vi "Shooter_Determiner.vi"() -> ()   [LabVIEW 2020]
uses:
  Subsystems/Cowl/Cowl_Cluster.ctl
  Subsystems/Cowl/Cowl_States.ctl
  <vilib>/Rock Robotics/WPI/DriverStation/WPI_DriverStationRobotMode2.ctl
  Subsystems/Flywheel/Flywheel_Cluster.ctl
  Subsystems/Flywheel/Flywheel_States.ctl
  Subsystems/Turret/Turret_Cluster.ctl
  Subsystems/Turret/Turret_States.ctl
  Shooter_Control_States.ctl
  Shooter_Cluster.ctl
  Globals/Turret_Globals.vi
  Globals/Flywheel_Globals.vi
  Globals/Cowl_Globals.vi
  Shooter_Globals.vi
  Robot Global Data.vi
  Globals/Sensor_Values.vi
panel:
  out "angle_to_target":dbl
  in  "Cowl_Puke_Goal_Angle":dbl=61.0
  in  "Flywheel_Puke_Velocity_Goal":dbl=1000.0
  in  "no_target_flywheel_velocity":dbl=3200.0
  in  "no_target_cowl_angle":dbl=61.0
  in  "disable turret auto_target":bool
  in  "use table in test":bool
  out "cowl_goal_angle":dbl=61.0
  out "Flywheel_Goal_Velocity":dbl=3200.0
  in  "use auto-target turret in test":bool
  in  "Cowl_Angle_Test_Goal":dbl=50.0
  in  "use front panel cowl goal":bool
  in  "use front panel flywheel velocity goal":bool
  in  "Flywheel_Velocity_Test_Goal":dbl=3500.0
  out "Limelight_Distance_To_Target (in)":dbl=124.83321913736278
  in  "Shooter_Table":dbl[][](array[numeric])=[[55.0, 3350.0, 60.0], [81.0, 3500.0, 54.0], [110.0, 3800.0, 50.0], [143.0, 4100.0, 45.0], [179.0, 4700.0, 43.0]]
  in  "Use Equation?":bool
  out "loop time":u32=31
  out "timed out?":bool=TRUE
  # "68    3800    61"
  # "distance | flywheel velocity | cowl angle"
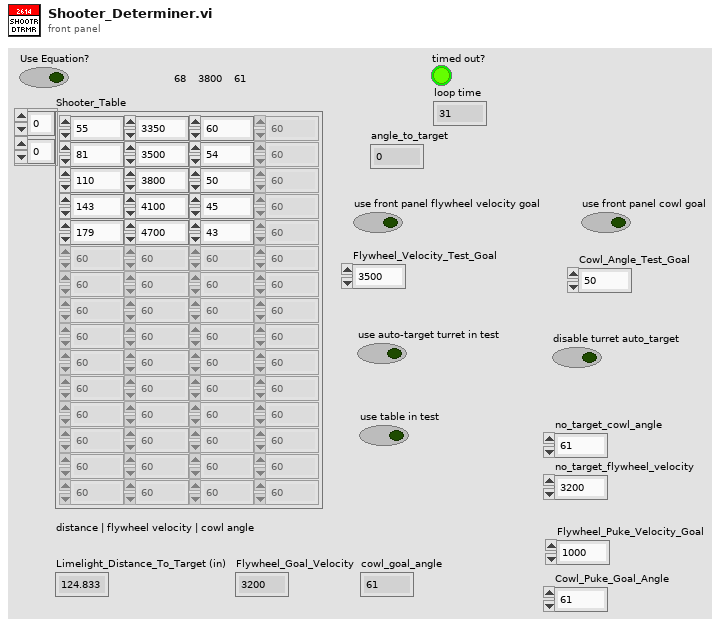
[diagram p1: front panel]
types:
  T1 = typedef "Shooter_Control_States.ctl" = enum16{"No-Op", "Limelight_Shooting", "Shoot_From_Pose", "Test", "Command_Shoot", "Manual", "Puke-Op", "Command_Shoot_From_Pose", "Turret Control", "Turret_Cowl_Zero"}
  T2 = typedef "Turret_Cluster.ctl" = cluster{"Turret_Control_State":T3, "Manual_Speed":dbl, "Step":i32, "Parameter_1":dbl, "Parameter_2":dbl, "Parameter_3":dbl, "Auto_Notifier":refnum<notifier>, "Goal_Angle":dbl, "Camera_Goal_X":dbl}
  T3 = typedef "Turret_States.ctl" = enum16{"Manual_Percent_Voltage", "Auto-Target", "Command_TurnToPosition", "Command_Auto_Target", "GoToZero", "No-Op", "Test_Position_Control", "Auto-Track"}
  T4 = typedef "Flywheel_Cluster.ctl" = cluster{"Flywheel_Throttle":dbl, "Flywheel_Control_State":T5, "Parameter_1":dbl, "Parameter_2":dbl, "Auto_Notifier":refnum<notifier>, "Step":dbl, "Flywheel_Velocity_Goal":dbl, "Flywheel_On ":bool}
  T5 = typedef "Flywheel_States.ctl" = enum16{"No-Op", "Percent_Voltage", "Speed_Control", "Speed_Control_Manual", "Command_SpinUp", "Command_SpinUpAuto"}
  T6 = typedef "WPI_DriverStationRobotMode2.ctl" = enum16{"Autonomous Disabled", "Autonomous Enabled", "Teleop Disabled", "Teleop Enabled", "Disconnected", "Finish", "Test Disabled", "Test Enabled", "Emergency Stopped"}
  T7 = typedef "Cowl_Cluster.ctl" = cluster{"Cowl_Control_State":T8, "Manual_Cowl_Throttle":dbl, "Cowl_Goal_Angle":dbl}
  T8 = typedef "Cowl_States.ctl" = enum16{"Manual_%VBus", "GoToAngle", "No-Op", "GoToZero"}
  T9 = typedef "Shooter_Cluster.ctl" = cluster{"Control_State":T1, "Shooting?":bool, "UpperGoal?":bool, "Limelight?":bool, "Flywheel_%Vbus":dbl, "Cowl_%Vbus":dbl, "Turret_%Vbus":dbl, "Parameters":dbl[], "Auto_Notifier":refnum<notifier>, "Step":i32, "Zero_Turret":bool, "Puke?":bool, "Turret_Target":dbl, "Turret_Control?":bool, "Turret_Manual_Control?":bool}
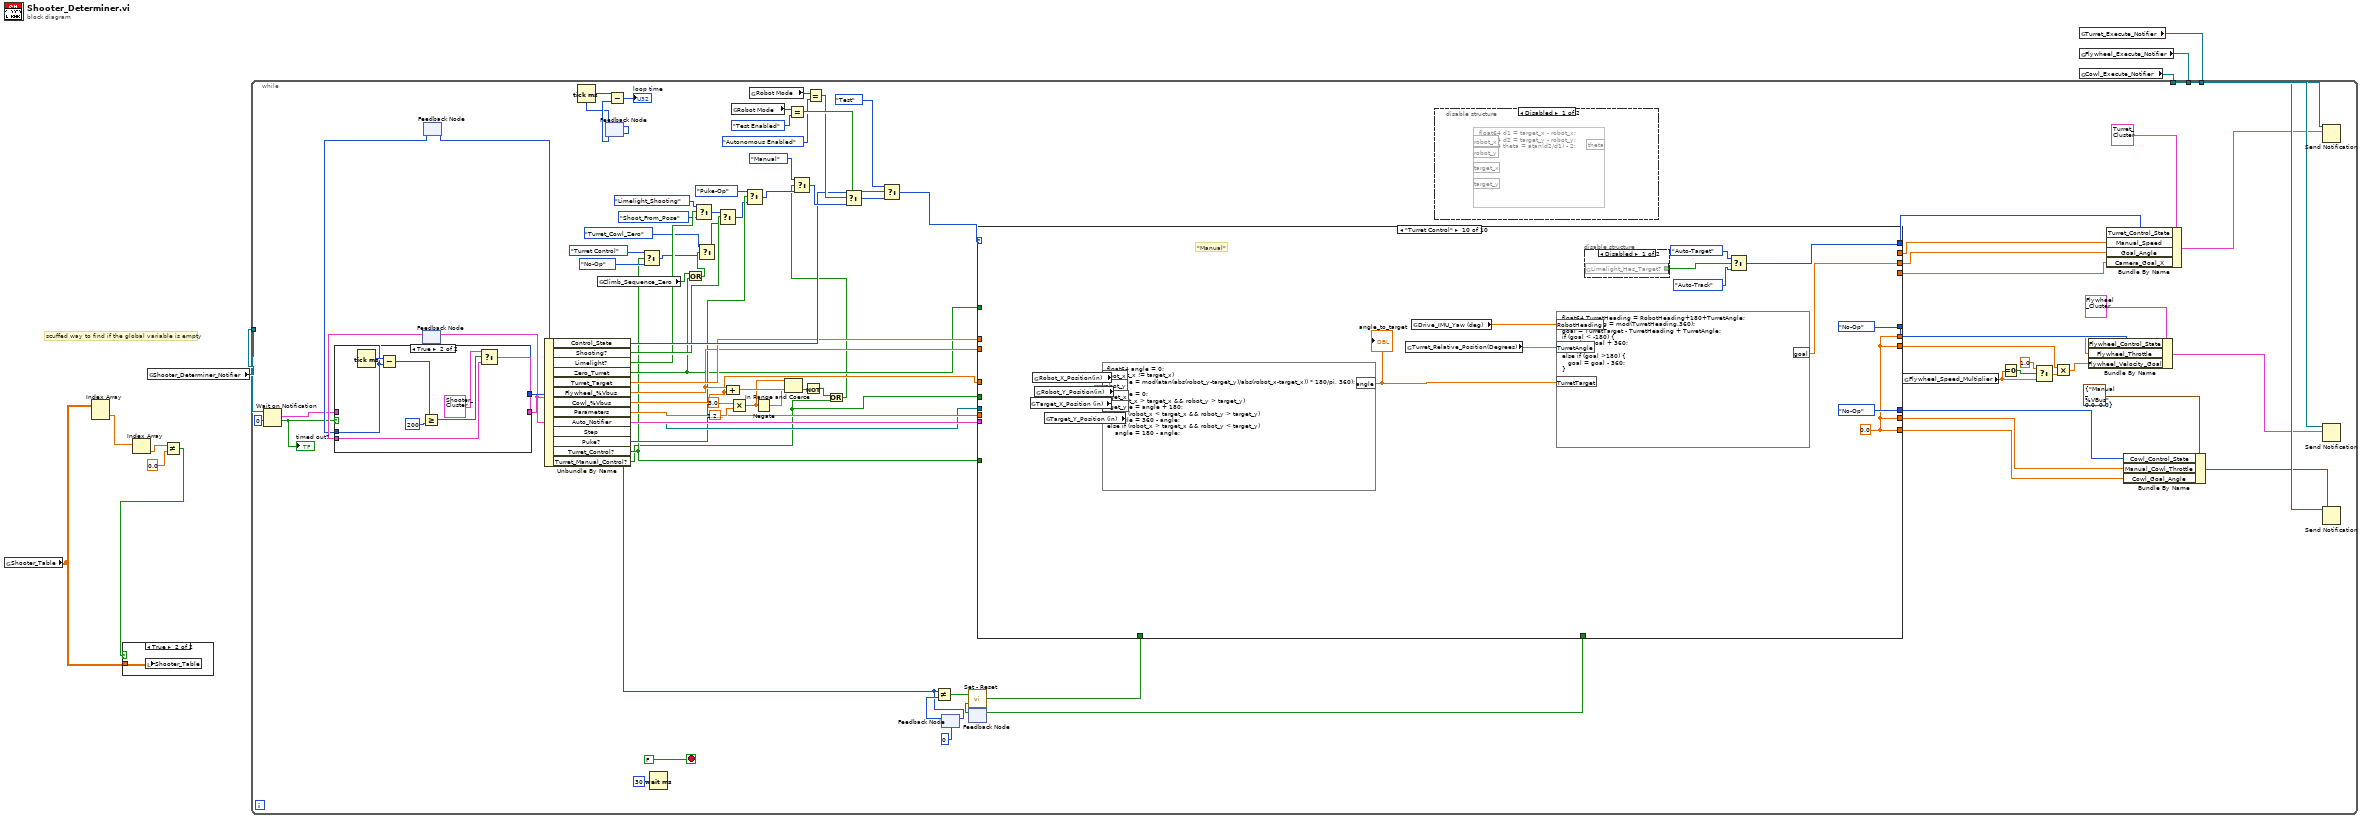
[diagram p0: block diagram]
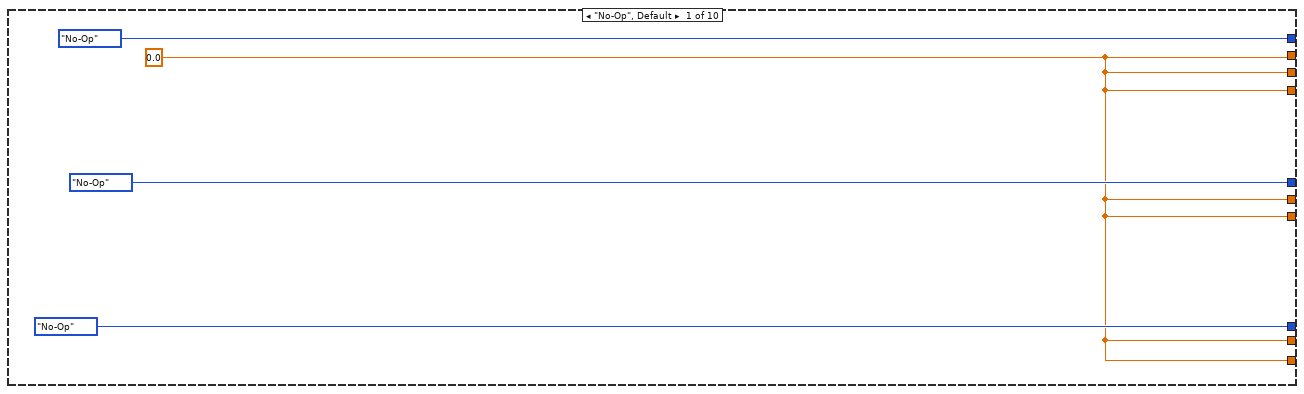
[diagram p4: hidden frame]
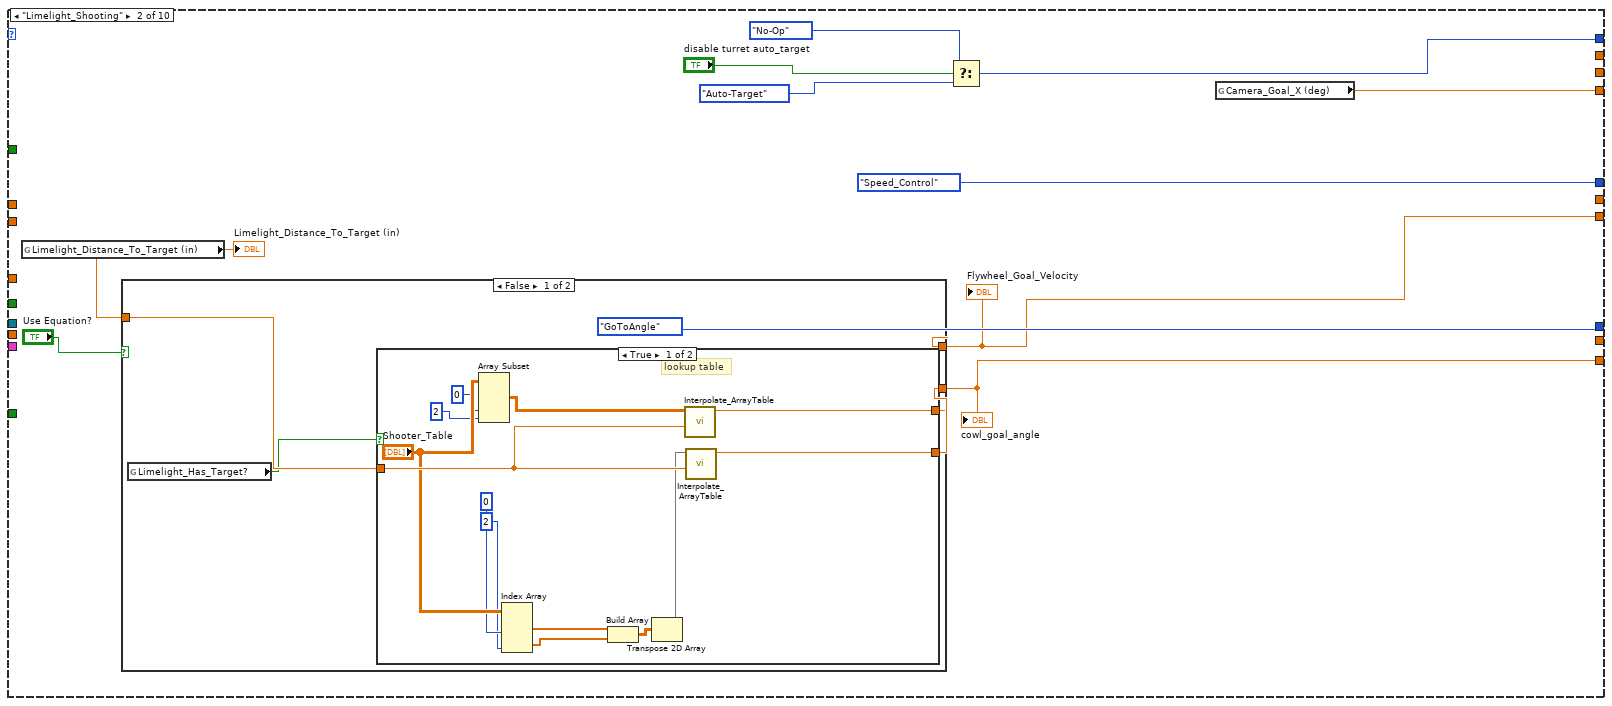
[diagram p5: hidden frame]
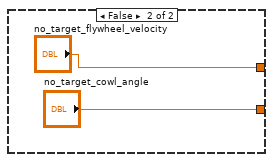
[diagram p6: hidden frame]
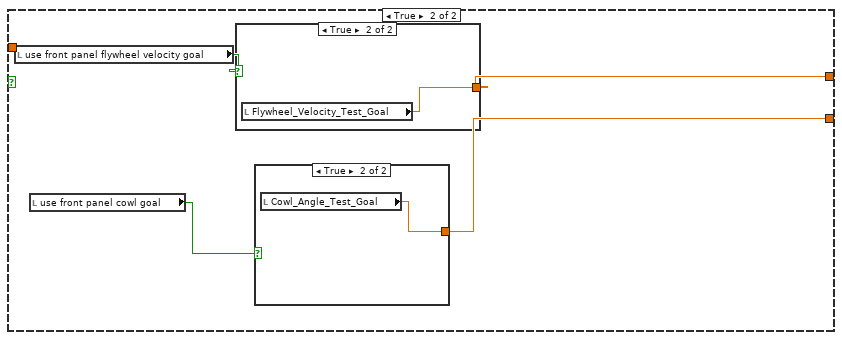
[diagram p7: hidden frame]
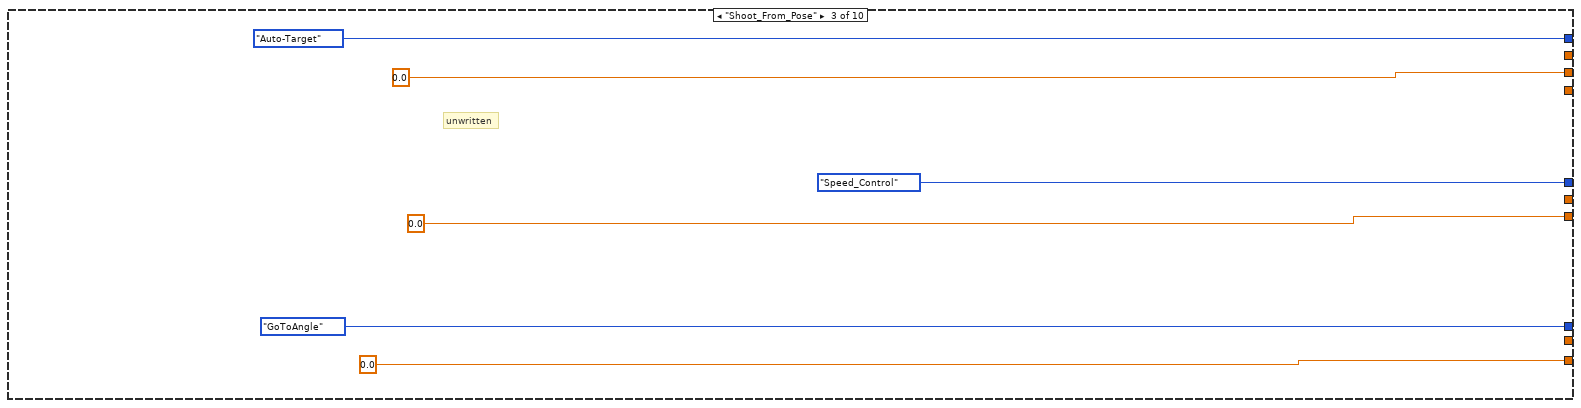
[diagram p10: hidden frame]
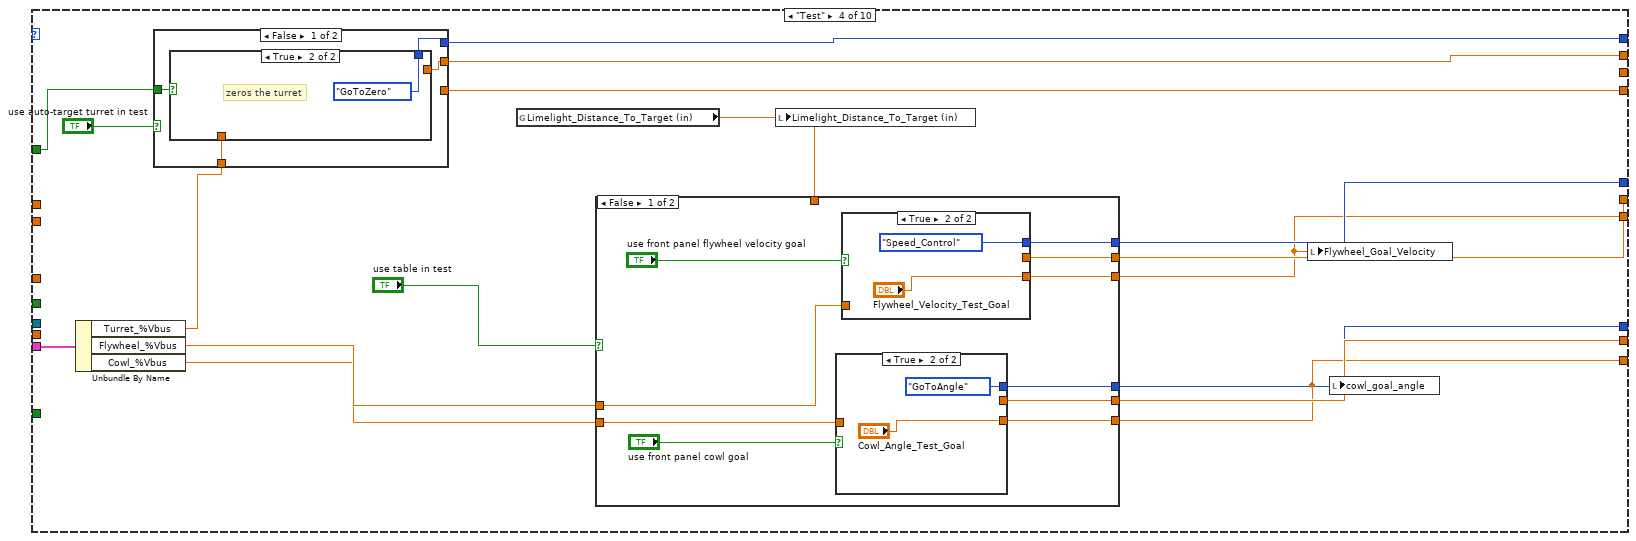
[diagram p11: hidden frame]
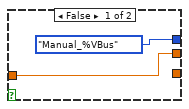
[diagram p12: hidden frame]
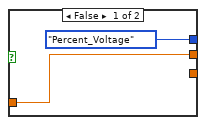
[diagram p13: hidden frame]
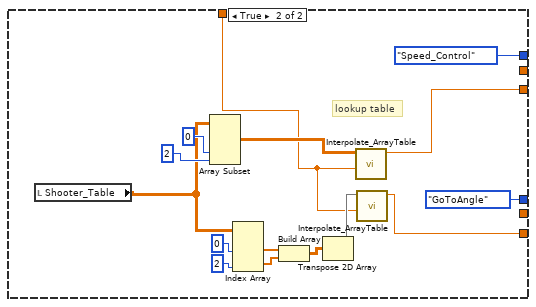
[diagram p14: hidden frame]
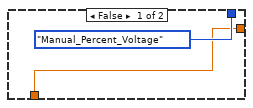
[diagram p15: hidden frame]
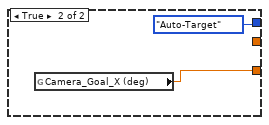
[diagram p16: hidden frame]
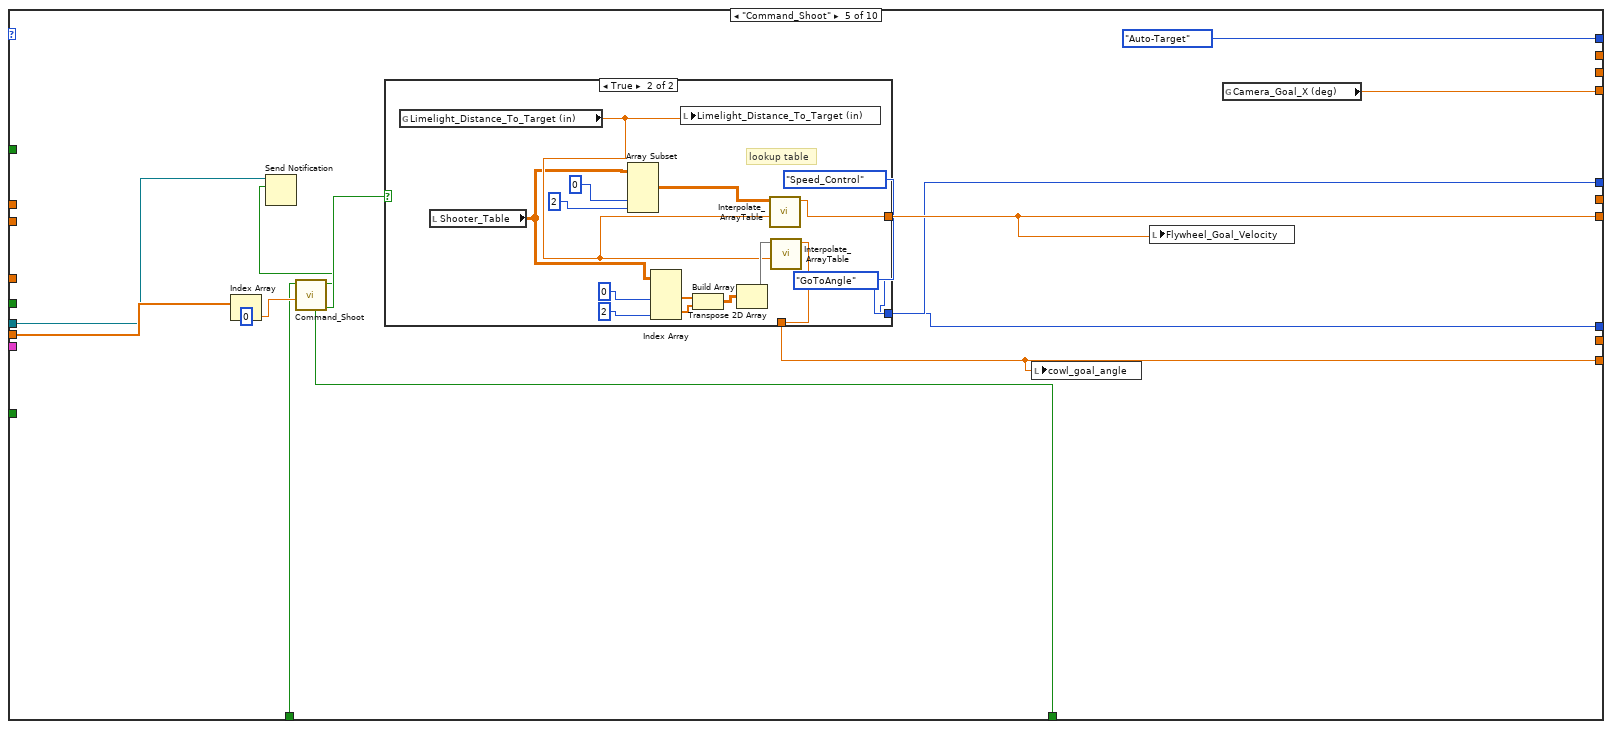
[diagram p17: hidden frame]
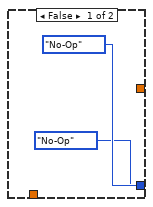
[diagram p18: hidden frame]
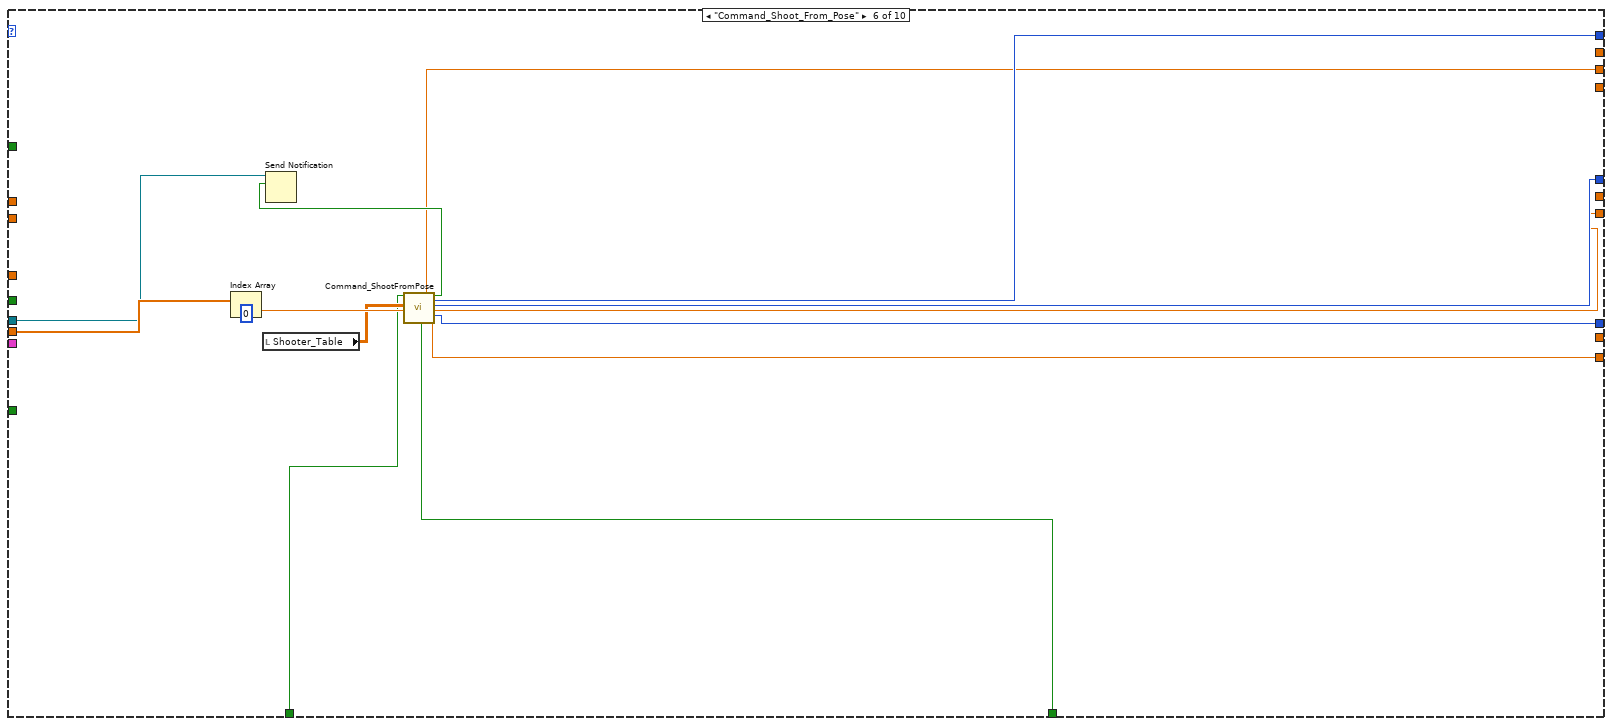
[diagram p19: hidden frame]
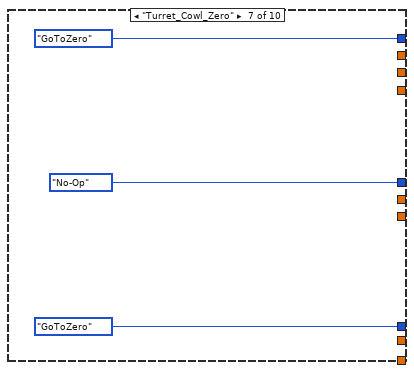
[diagram p20: hidden frame]
diagram:
  # "scuffed way to find if the global variable is empty"
  n1 = global read "Shooter_Globals.vi" "Shooter_Table"() -> (w6:dbl[][])
  n2 = Index Array(array=w6) -> (element=w5:dbl[])  [unwired: 2 in]
  n3 = Index Array(array=w5) -> (element=w4:dbl)  [unwired: 1 in]
  n4 = global read "Shooter_Globals.vi" "Shooter_Determiner_Notifier"() -> (w1:refnum<notifier>)
  n5 = Not Equal?(x=w4, y=0.0) -> (x != y?=w3:bool)
  n6 = case shown="True" w3 {
    tunnel: w6 -> [_ w10]
    frame False {
    }
    frame True {
      n7 = local write "Shooter_Table"(w10) -> ()
    }
  }
  n8 = global read "Turret_Globals.vi" "Turret_Execute_Notifier"() -> (w9:refnum<notifier>)
  n9 = global read "Flywheel_Globals.vi" "Flywheel_Execute_Notifier"() -> (w8:refnum<notifier>)
  n10 = global read "Cowl_Globals.vi" "Cowl_Execute_Notifier"() -> (w7:refnum<notifier>)
  n11 = while {
    tunnel: w1 -> [w98]
    tunnel: w9 -> [w89]
    tunnel: w8 -> [w91]
    tunnel: w7 -> [w90]
    stop <- FALSE stop-if-true
    n12 = Wait on Notification(notifier=w98, timeout in ms (-1)=0) -> (notification=w73:T9, timed out?=w72:bool)  [unwired: 2 in, 2 out]
    "timed out?" <- w72
    n13 = feedback #1() -> (w76:T9)  [unwired: 1 in]
    n14 = feedback #2() -> (w74:u32)  [unwired: 1 in]
    n15 = case shown="True" w72 {
      tunnel: w73 -> [w297 _]
      tunnel: [w297 w306] -> w71
      tunnel: w76 -> [_ w305]
      tunnel: [w298 w303] -> w75
      tunnel: w74 -> [_ w303]
      frame False {
        n16 = Tick Count (ms)() -> (millisecond timer value=w298:u32)
      }
      frame True {
        n17 = Tick Count (ms)() -> (millisecond timer value=w304:u32)
        n18 = Subtract(x=w304, y=w303) -> (x-y=w301:u32)
        n19 = Greater Or Equal?(x=w301, y=u32 200) -> (x >= y?=w302:bool)
        n20 = Select(t=T9 {"Control_State"=enum."No-Op", "Shooting?"=FALSE, "UpperGoal?"=FALSE, "Limelight?"=FALSE, "Flywheel_%Vbus"=0.0, "Cowl_%Vbus"=0.0, "Turret_%Vbus"=0.0, "Parameters"=[], "Auto_Notifier"=refnum, "Step"=0, "Zero_Turret"=FALSE, "Puke?"=FALSE, "Turret_Target"=0.0, "Turret_Control?"=FALSE, "Turret_Manual_Control?"=FALSE} ("notification"), s=w302, f=w305) -> (s? t:f=w306:T9)
      }
    }
    n21 = feedback-in #1(w71) -> ()
    n22 = feedback-in #2(w75) -> ()
    n23 = Unbundle By Name(w71) -> ("Control_State"=w45:T1, "Shooting?"=w44:bool, "Limelight?"=w43:bool, "Zero_Turret"=w21:bool, "Turret_Target"=w42:dbl, "Flywheel_%Vbus"=w41:dbl, "Cowl_%Vbus"=w40:dbl, "Parameters"=w39:dbl[], "Auto_Notifier"=w38:refnum<notifier>, "Step"=w37:i32, "Puke?"=w36:bool, "Turret_Control?"=w14:bool, "Turret_Manual_Control?"=w11:bool)
    n24 = Tick Count (ms)() -> (millisecond timer value=w79:u32)
    n25 = global read "Shooter_Globals.vi" "Climb_Sequence_Zero"() -> (w20:bool)
    n26 = feedback-in #3(w79) -> ()
    n27 = feedback #3() -> (w80:u32)  [unwired: 1 in]
    n28 = Subtract(x=w79, y=w80) -> (x-y=→"loop time":u32)
    n29 = Select(t=Shooter_Control_States."Turret Control" ("Control_State"), s=w14, f=Shooter_Control_States."No-Op" ("Control_State")) -> (s? t:f=w19:T1)
    n30 = Wait (ms)(milliseconds to wait=u32 30) -> ()  [unwired: 1 out]
    n31 = Or(x=w20, y=w21) -> (x .or. y?=w22:bool)
    n32 = Select(t=Shooter_Control_States."Limelight_Shooting" ("Control_State"), s=w43, f=Shooter_Control_States."Shoot_From_Pose" ("Control_State")) -> (s? t:f=w55:T1)
    n33 = Select(t=Shooter_Control_States."Turret_Cowl_Zero" ("Control_State"), s=w22, f=w19) -> (s? t:f=w24:T1)
    n34 = Select(t=w55, s=w44, f=w24) -> (s? t:f=w35:T1)
    n35 = Compound Arithmetic op=ADD(w41, w40) -> (w54:dbl)
    n36 = Multiply(x=3.0, y=2.220446049250313e-16) -> (x*y=w51:dbl)
    n37 = global read "Robot Global Data.vi" "Robot Mode"() -> (w84:T6)
    n38 = Select(t=Shooter_Control_States."Puke-Op", s=w36, f=w35) -> (s? t:f=w23:T1)
    n39 = global read "Robot Global Data.vi" "Robot Mode"() -> (w67:T6)
    n40 = Negate(x=w51) -> (-x=w52:dbl)
    n41 = In Range and Coerce(upper limit=w51, x=w54, lower limit=w52) -> (In Range?=w53:bool)  [unwired: 1 out]
    n42 = Equal?(x=w84, y=WPI_DriverStationRobotMode2."Test Enabled" ("Robot Mode")) -> (x = y?=w82:bool)
    n43 = Not(x=w53) -> (.not. x?=w13:bool)
    n44 = Equal?(x=w67, y=WPI_DriverStationRobotMode2."Autonomous Enabled" ("Robot Mode")) -> (x = y?=w66:bool)
    n45 = Or(x=w13, y=w11) -> (x .or. y?=w12:bool)
    n46 = Select(t=Shooter_Control_States."Manual", s=w12, f=w23) -> (s? t:f=w56:T1)
    n47 = Select(t=w45, s=w66, f=w56) -> (s? t:f=w65:T1)
    n48 = Select(t=Shooter_Control_States."Test" ("Control_State"), s=w82, f=w65) -> (s? t:f=w83:T1)
    n49 = feedback #4(0 ("Step")) -> (w62:i32)
    n50 = Not Equal?(x=w37, y=w62) -> (x != y?=w63:bool)
    n51 = feedback-in #4(w37) -> ()
    n52 = feedback #5() -> (w64:bool)  [unwired: 1 in]
    n53 = call "Set - Reset.vi"("Reset"=w64, "Set"=w63) -> ("Output"=w59:bool)
    n54 = case shown="\"Turret Control\"" w83 {
      tunnel: [Flywheel_States."No-Op" ("Control_States") Flywheel_States."Speed_Control" ("Flywheel_Control_State") Flywheel_States."Speed_Control" ("Flywheel_Control_State") w159 w205 w239 Flywheel_States."No-Op" ("Control_States") w261 Flywheel_States."Speed_Control" ("Control_States") Flywheel_States."No-Op" ("Control_States")] -> w93
      tunnel: [Turret_States."No-Op" ("Control_State") w103 Turret_States."Auto-Target" ("Control_State") w157 Turret_States."Auto-Target" ("Control_State") w240 Turret_States."GoToZero" ("Control_State") w262 Turret_States."No-Op" ("Control_State") w281] -> w48
      tunnel: [Cowl_States."No-Op" ("Control_State") Cowl_States."GoToAngle" ("Cowl_Control_State") Cowl_States."GoToAngle" ("Cowl_Control_State") w154 w204 w238 Cowl_States."GoToZero" ("Cowl_Control_State") w260 Cowl_States."GoToAngle" ("Cowl_Control_State") Cowl_States."No-Op" ("Cowl_Control_State")] -> w47
      tunnel: w21 -> [_ _ _ w145 _ _ _ _ _ _]
      tunnel: [w99 _ 0.0 _ _ w236 _ w258 _ w292] -> w25
      tunnel: [w99 _ _ w158 _ _ _ w252 _ w293] -> w92
      tunnel: [w99 _ _ w155 _ _ _ w259 _ w293] -> w95
      tunnel: [w99 w107 0.0 w149 w213 w237 _ _ "Cowl_Puke_Goal_Angle" w293] -> w94
      tunnel: [w99 _ _ w151 _ _ _ _ _ _] -> w77
      tunnel: [w99 w108 0.0 w148 w214 w235 _ 0.0 ("Cowl_Puke_Goal_Angle") "Flywheel_Puke_Velocity_Goal" w293] -> w31
      tunnel: w71 -> [_ _ _ w161 _ _ _ _ _ _]
      tunnel: [w99 w111 _ w150 w215 _ _ _ _ _] -> w69
      tunnel: w42 -> [_ _ _ _ _ _ _ w257 _ _]
      tunnel: w39 -> [_ _ _ _ w217 w248 _ _ _ _]
      tunnel: [_ _ _ _ w210 w241 _ _ _ _] -> w60
      tunnel: w59 -> [_ _ _ _ w209 w242 _ _ _ _]
      tunnel: w38 -> [_ _ _ _ w206 w246 _ _ _ _]
      tunnel: w40 -> [_ _ _ _ _ _ _ w254 _ _]
      tunnel: w41 -> [_ _ _ _ _ _ _ w255 _ _]
      tunnel: w14 -> [_ _ _ _ _ _ _ _ _ _]
      tunnel: w11 -> [_ _ _ _ _ _ _ w256 _ _]
      frame "No-Op", Default {
        w99 = 0.0
      }
      frame "Limelight_Shooting" {
        n55 = global read "Sensor_Values.vi" "Limelight_Distance_To_Target (in)"() -> (w109:dbl)
        "Limelight_Distance_To_Target (in)" <- w109
        n56 = case shown="False" "Use Equation?" {
          tunnel: w109 -> [w116 _]
          tunnel: [w115 w135] -> w108
          tunnel: [w117 w134] -> w107
          frame False {
            n57 = global read "Sensor_Values.vi" "Limelight_Has_Target?"() -> (w114:bool)
            n58 = case shown="True" w114 {
              tunnel: w116 -> [w129 _]
              tunnel: [w128 "no_target_flywheel_velocity"] -> w115
              tunnel: [w130 "no_target_cowl_angle"] -> w117
              frame True {
                # "lookup table"
                n59 = Array Subset(array="Shooter_Table", index (col)=0 ("index"), length (col)=2 ("length")) -> (w127:dbl[][])  [unwired: 2 in]
                n60 = Index Array(array="Shooter_Table", index (col) #1=0 ("index (row)"), index (col) #2=2 ("index (row)")) -> (element #1=w125:dbl[], element #2=w124:dbl[])  [unwired: 2 in]
                n61 = Build Array(w125, w124) -> (w121:dbl[][])
                n62 = Transpose 2D Array(2D array=w121) -> (transposed array=w120:dbl[][])
                n63 = call "Interpolate_ArrayTable.vi"("Desired_Distance"=w129, "array"=w127) -> ("RPM"=w128:dbl)  [unwired: 9 in]
                n64 = call "Interpolate_ArrayTable.vi"("Desired_Distance"=w129, "array"=w120) -> ("RPM"=w130:dbl)  [unwired: 9 in]
              }
              frame False {
              }
            }
          }
          frame True {
            n65 = local read "use front panel flywheel velocity goal"() -> (w136:bool)
            n66 = local read "use front panel cowl goal"() -> (w133:bool)
            n67 = case shown="True" w136 {
              tunnel: [_ w138] -> w135
              frame False {
              }
              frame True {
                n68 = local read "Flywheel_Velocity_Test_Goal"() -> (w138:dbl)
              }
            }
            n69 = case shown="True" w133 {
              tunnel: [_ w137] -> w134
              frame False {
              }
              frame True {
                n70 = local read "Cowl_Angle_Test_Goal"() -> (w137:dbl)
              }
            }
          }
        }
        "Flywheel_Goal_Velocity" <- w108
        "cowl_goal_angle" <- w107
        n71 = Select(t=Turret_States."No-Op", s="disable turret auto_target", f=Turret_States."Auto-Target" ("Control_State")) -> (s? t:f=w103:T3)
        n72 = global read "Sensor_Values.vi" "Camera_Goal_X (deg)"() -> (w111:dbl)
      }
      frame "Shoot_From_Pose" {
        # "unwritten"
      }
      frame "Test" {
        n73 = Unbundle By Name(w161) -> ("Turret_%Vbus"=w152:dbl, "Flywheel_%Vbus"=w160:dbl, "Cowl_%Vbus"=w156:dbl)
        n74 = case shown="False" "use auto-target turret in test" {
          tunnel: [w198 Turret_States."Auto-Target" ("Control_State")] -> w157
          tunnel: w145 -> [w197 _]
          tunnel: w152 -> [w196 _]
          tunnel: [w195 _] -> w151
          tunnel: [_ w202] -> w150
          frame False {
            n75 = case shown="True" w197 {
              tunnel: [Turret_States."Manual_Percent_Voltage" ("Control_State") Turret_States."GoToZero" ("Control_State")] -> w198
              tunnel: w196 -> [w199 _]
              tunnel: [w199 _] -> w195
              frame False {
              }
              frame True {
                # "zeros the turret"
              }
            }
          }
          frame True {
            n76 = global read "Sensor_Values.vi" "Camera_Goal_X (deg)"() -> (w202:dbl)
          }
        }
        n77 = global read "Sensor_Values.vi" "Limelight_Distance_To_Target (in)"() -> (w146:dbl)
        n78 = case shown="False" "use table in test" {
          tunnel: w160 -> [w171 _]
          tunnel: [w170 Flywheel_States."Speed_Control" ("Control_States")] -> w159
          tunnel: [w169 w183] -> w148
          tunnel: [w167 _] -> w158
          tunnel: w156 -> [w166 _]
          tunnel: [w164 _] -> w155
          tunnel: [w163 Cowl_States."GoToAngle" ("Cowl_Control_State")] -> w154
          tunnel: [w162 w184] -> w149
          tunnel: w146 -> [_ w180]
          frame False {
            n79 = case shown="True" "use front panel cowl goal" {
              tunnel: w166 -> [w173 _]
              tunnel: [w173 _] -> w164
              tunnel: [Cowl_States."Manual_%VBus" ("Cowl_Control_State") Cowl_States."GoToAngle" ("Cowl_Control_State")] -> w163
              tunnel: [_ "Cowl_Angle_Test_Goal"] -> w162
              frame False {
              }
              frame True {
              }
            }
            n80 = case shown="True" "use front panel flywheel velocity goal" {
              tunnel: w171 -> [w177 _]
              tunnel: [w177 _] -> w167
              tunnel: [Flywheel_States."Percent_Voltage" ("Control_States") Flywheel_States."Speed_Control" ("Control_States")] -> w170
              tunnel: [_ "Flywheel_Velocity_Test_Goal"] -> w169
              frame False {
              }
              frame True {
              }
            }
          }
          frame True {
            # "lookup table"
            n81 = local read "Shooter_Table"() -> (w185:dbl[][])
            n82 = Array Subset(array=w185, index (col)=0 ("index"), length (col)=2 ("length")) -> (w194:dbl[][])  [unwired: 2 in]
            n83 = Index Array(array=w185, index (col) #1=0 ("index (row)"), index (col) #2=2 ("index (row)")) -> (element #1=w193:dbl[], element #2=w192:dbl[])  [unwired: 2 in]
            n84 = Build Array(w193, w192) -> (w187:dbl[][])
            n85 = Transpose 2D Array(2D array=w187) -> (transposed array=w186:dbl[][])
            n86 = call "Interpolate_ArrayTable.vi"("Desired_Distance"=w180, "array"=w194) -> ("RPM"=w183:dbl)  [unwired: 9 in]
            n87 = call "Interpolate_ArrayTable.vi"("Desired_Distance"=w180, "array"=w186) -> ("RPM"=w184:dbl)  [unwired: 9 in]
          }
        }
        n88 = local write "Limelight_Distance_To_Target (in)"(w146) -> ()
        n89 = local write "Flywheel_Goal_Velocity"(w148) -> ()
        n90 = local write "cowl_goal_angle"(w149) -> ()
      }
      frame "Command_Shoot" {
        n91 = Index Array(array=w217, index=0) -> (element=w211:dbl)
        n92 = call "Command_Shoot.vi"("Startup"=w209, "Timeout"=w211) -> ("Reint"=w210:bool, "Completed"=w207:bool, "Output"=w208:bool)  [unwired: 6 in]
        n93 = Send Notification(notification=w207, notifier=w206) -> ()  [unwired: 1 in, 2 out]
        n94 = case shown="True" w208 {
          tunnel: [_ w224] -> w214
          tunnel: [_ w223] -> w213
          tunnel: [Flywheel_States."No-Op" ("Control_States") Flywheel_States."Speed_Control" ("Control_States")] -> w205
          tunnel: [Cowl_States."No-Op" ("Cowl_Control_State") Cowl_States."GoToAngle" ("Cowl_Control_State")] -> w204
          frame False {
          }
          frame True {
            # "lookup table"
            n95 = global read "Sensor_Values.vi" "Limelight_Distance_To_Target (in)"() -> (w225:dbl)
            n96 = local read "Shooter_Table"() -> (w222:dbl[][])
            n97 = Array Subset(array=w222, index (col)=0 ("index"), length (col)=2 ("length")) -> (w234:dbl[][])  [unwired: 2 in]
            n98 = Index Array(array=w222, index (col) #1=0 ("index (row)"), index (col) #2=2 ("index (row)")) -> (element #1=w233:dbl[], element #2=w232:dbl[])  [unwired: 2 in]
            n99 = local write "Limelight_Distance_To_Target (in)"(w225) -> ()
            n100 = Build Array(w233, w232) -> (w227:dbl[][])
            n101 = Transpose 2D Array(2D array=w227) -> (transposed array=w226:dbl[][])
            n102 = call "Interpolate_ArrayTable.vi"("Desired_Distance"=w225, "array"=w234) -> ("RPM"=w224:dbl)  [unwired: 9 in]
            n103 = call "Interpolate_ArrayTable.vi"("Desired_Distance"=w225, "array"=w226) -> ("RPM"=w223:dbl)  [unwired: 9 in]
          }
        }
        n104 = local write "cowl_goal_angle"(w213) -> ()
        n105 = local write "Flywheel_Goal_Velocity"(w214) -> ()
        n106 = global read "Sensor_Values.vi" "Camera_Goal_X (deg)"() -> (w215:dbl)
      }
      frame "Command_Shoot_From_Pose" {
        n107 = Index Array(array=w248, index=0) -> (element=w245:dbl)
        n108 = local read "Shooter_Table"() -> (w244:dbl[][])
        n109 = call "Command_ShootFromPose.vi"("Startup"=w242, "Shooter_table"=w244, "Timeout"=w245) -> ("Reint"=w241:bool, "turret_angle(deg)"=w236:dbl, "Completed"=w243:bool, "turret_state"=w240:T3, "flywheel_state"=w239:T5, "flywheel_speed(RPM)"=w235:dbl, "cowl_state"=w238:T8, "cowl_angle(deg)"=w237:dbl)  [unwired: 9 in]
        n110 = Send Notification(notification=w243, notifier=w246) -> ()  [unwired: 1 in, 2 out]
      }
      frame "Turret_Cowl_Zero" {
      }
      frame "Manual" {
        # "\"Manual\""
        n111 = case shown="False" w256 {
          tunnel: [Turret_States."No-Op" ("Control_State") Turret_States."Auto-Track" ("Control_State")] -> w262
          tunnel: [Flywheel_States."Percent_Voltage" ("Control_States") Flywheel_States."No-Op" ("Control_States")] -> w261
          tunnel: [Cowl_States."Manual_%VBus" ("Cowl_Control_State") Cowl_States."No-Op" ("Cowl_Control_State")] -> w260
          tunnel: [w265 w268] -> w259
          tunnel: [_ w270] -> w258
          tunnel: w257 -> [_ w269]
          tunnel: w255 -> [w263 _]
          tunnel: w254 -> [w265 _]
          tunnel: [w263 w268] -> w252
          frame False {
          }
          frame True {
            w268 = 0.0 ("Cowl_Puke_Goal_Angle")
            n112 = global read "Sensor_Values.vi" "Turret_Relative_Position(Degrees)"() -> (w275:dbl)
            n113 = global read "Sensor_Values.vi" "Drive_IMU_Yaw (deg)"() -> (w274:dbl)
            n114 = formula code="float64 TurretHeading = RobotHeading+180+TurretAngle;\nTurretHeading = mod(TurretHeading,360);\ngoal = TurretTarget - TurretHeading + TurretAngle;\nif (goal < -180) {\n   goal = goal + 360;\n} \nelse if (goal >180) {\n   goal = goal - 360;\n}"("TurretAngle"=w275, "RobotHeading"=w274, "TurretTarget"=w269) -> ("goal"=w270:dbl)
          }
        }
      }
      frame "Puke-Op" {
      }
      frame "Turret Control" {
        w293 = 0.0 ("Cowl_Puke_Goal_Angle")
        # "\"Manual\""
        n115 = global read "Shooter_Globals.vi" "Target_X_Position (in)"() -> (w287:dbl)
        n116 = global read "Sensor_Values.vi" "Robot_X_Position(in)"() -> (w289:dbl)
        n117 = global read "Sensor_Values.vi" "Robot_Y_Position(in)"() -> (w290:dbl)
        n118 = global read "Shooter_Globals.vi" "Target_Y_Position (in)"() -> (w288:dbl)
        n119 = formula code="float64 angle = 0;\nif(robot_x != target_x)\n    angle = mod(atan(abs(robot_y-target_y)/abs(robot_x-target_x)) * 180/pi, 360);\nelse\n    angle = 0;\nif (robot_x > target_x && robot_y > target_y)\n    angle = angle + 180;\nelse if (robot_x < target_x && robot_y > target_y)\n    angle = 360 - angle;\nelse if (robot_x > target_x && robot_y < target_y)\n    angle = 180 - angle;"("robot_x"=w289, "robot_y"=w290, "target_x"=w287, "target_y"=w288) -> ("angle"=w291:dbl)
        "angle_to_target" <- w291
        n120 = global read "Sensor_Values.vi" "Turret_Relative_Position(Degrees)"() -> (w286:dbl)
        n121 = global read "Sensor_Values.vi" "Drive_IMU_Yaw (deg)"() -> (w285:dbl)
        n122 = formula code="float64 TurretHeading = RobotHeading+180+TurretAngle;\nTurretHeading = mod(TurretHeading,360);\ngoal = TurretTarget - TurretHeading + TurretAngle;\nif (goal < -180) {\n   goal = goal + 360;\n} \nelse if (goal >180) {\n   goal = goal - 360;\n}"("TurretAngle"=w286, "RobotHeading"=w285, "TurretTarget"=w291) -> ("goal"=w292:dbl)
        n123 = disable-structure shown="Disabled" {
          disable-tunnel: [w296 _] -> w282
          frame Disabled {
            n124 = global read "Sensor_Values.vi" "Limelight_Has_Target?"() -> (w296:bool)
          }
          frame Enabled {
          }
        }
        n125 = Select(t=Turret_States."Auto-Target" ("Control_State"), s=w282, f=Turret_States."Auto-Track" ("Control_State")) -> (s? t:f=w281:T3)
      }
    }
    n126 = feedback-in #5(w60) -> ()
    n127 = disable-structure shown="Disabled" {
      frame Disabled {
        n128 = formula code="float64 d1 = target_x - robot_x;\nfloat64 d2 = target_y - robot_y; \nfloat64 theta = atan(d2/d1) - 2;"() -> ()  [unwired: 4 in, 1 out]
      }
      frame Enabled {
      }
    }
    n129 = global read "Shooter_Globals.vi" "Flywheel_Speed_Multiplier"() -> (w27:dbl)
    n130 = Equal To 0?(x=w27) -> (x = 0?=w29:bool)
    n131 = Select(t=1.0, s=w29, f=w27) -> (s? t:f=w26:dbl)
    n132 = Multiply(x=w31, y=w26) -> (x*y=w30:dbl)
    n133 = Bundle By Name(cluster=T4 {"Flywheel_Throttle"=0.0, "Flywheel_Control_State"=enum."No-Op", "Parameter_1"=0.0, "Parameter_2"=0.0, "Auto_Notifier"=refnum, "Step"=0.0, "Flywheel_Velocity_Goal"=0.0, "Flywheel_On "=FALSE} ("Flywheel_Cluster"), "Flywheel_Control_State"=w93, "Flywheel_Throttle"=w92, "Flywheel_Velocity_Goal"=w30) -> (w87:T4)
    n134 = Bundle By Name(cluster=T2 {"Turret_Control_State"=enum."Manual_Percent_Voltage", "Manual_Speed"=0.0, "Step"=0, "Parameter_1"=0.0, "Parameter_2"=0.0, "Parameter_3"=0.0, "Auto_Notifier"=refnum, "Goal_Angle"=0.0, "Camera_Goal_X"=0.0} ("Turret_Cluster"), "Turret_Control_State"=w48, "Manual_Speed"=w77, "Goal_Angle"=w25, "Camera_Goal_X"=w69) -> (w88:T2)
    n135 = Bundle By Name(cluster=T7 {"Cowl_Control_State"=enum."Manual_%VBus", "Manual_Cowl_Throttle"=0.0, "Cowl_Goal_Angle"=0.0} ("Cowl_Cluster"), "Cowl_Control_State"=w47, "Manual_Cowl_Throttle"=w95, "Cowl_Goal_Angle"=w94) -> (w86:T7)
    n136 = Send Notification(notification=w88, notifier=w89) -> ()  [unwired: 1 in, 2 out]
    n137 = Send Notification(notification=w87, notifier=w91) -> ()  [unwired: 1 in, 2 out]
    n138 = Send Notification(notification=w86, notifier=w90) -> ()  [unwired: 1 in, 2 out]
  }
